vi "READ_xlsx.vi"(2 "该文档引用输入":refnum<k7>, 3 "错误输入（无错误）":errorcluster) -> (0 "文档内容输出":string[][](array[string]), 1 "错误输出":errorcluster)   [LabVIEW 2014]
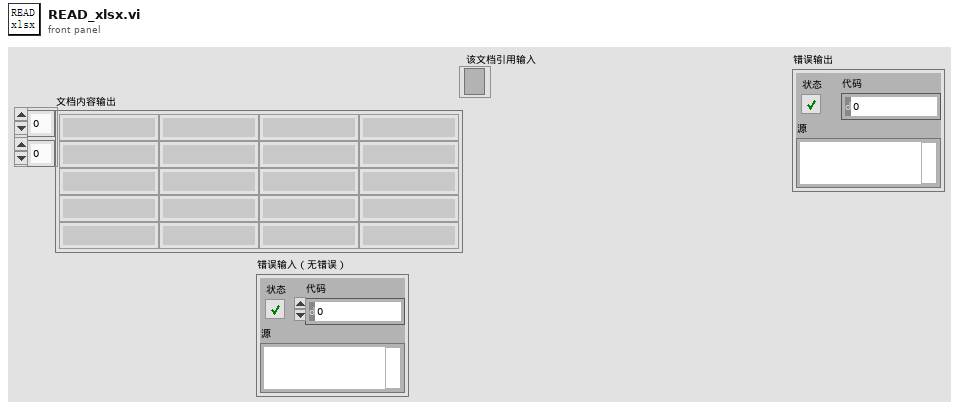
[diagram p1: front panel]
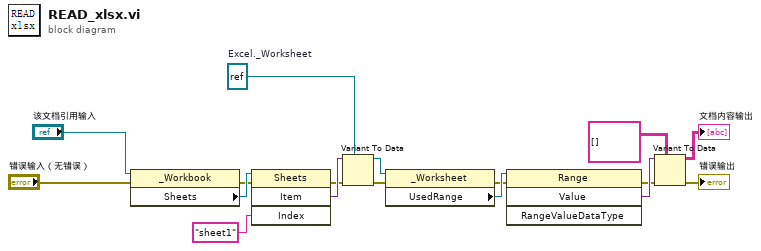
[diagram p0: block diagram]
diagram:
  w14 = refnum<k7> refnum  # Excel._Worksheet
  n1 = property class="_Workbook"(reference="该文档引用输入", error in="错误输入（无错误）") -> (error out=w12:errorcluster, "Sheets"=w17:refnum<k7>)  [unwired: 1 out]
  n2 = invoke class="Sheets" method="Item"(reference=w17, error in=w12, "Index"="sheet1" ("字符串")) -> (error out=w13:errorcluster, "Item"=w15:variant)  [unwired: 1 in, 2 out]
  n3 = Variant To Data(error in=w13, type=w14, Variant=w15) -> (data=w11:refnum<k7>, error out=w10:errorcluster)
  n4 = property class="_Worksheet"(reference=w11, error in=w10) -> (error out=w8:errorcluster, "UsedRange"=w9:refnum<k7>)  [unwired: 1 out]
  n5 = invoke class="Range" method="Value"(reference=w9, error in=w8) -> (error out=w6:errorcluster, "Value"=w7:variant)  [unwired: 2 in, 2 out]
  n6 = Variant To Data(error in=w6, type=string[][] [] ("数组"), Variant=w7) -> (data=→"文档内容输出":string[][], error out=→"错误输出":errorcluster)
